vi "Write Current.vi"(8 "error in":errorcluster, 10 "Current":dbl, 11 "69X_79X in":refnum<class "7976A.lvclass">) -> (0 "error out":errorcluster, 3 "69X_79X out":refnum<class "7976A.lvclass">)   [LabVIEW 2019, in "7976A.lvlib" / "7976A.lvclass"]
uses:
  Library/7976A.lvclass
  C:/Users/Public/Documents/Development/builds/Instruments/PowerSupply.lvlibp/Library/PowerSupply.lvclass
  Library/7976A.lvclass/7976A.ctl
  Read Local Resource.vi
  builds/Instruments/PowerSupply.lvlibp/Library/PowerSupply.lvclass
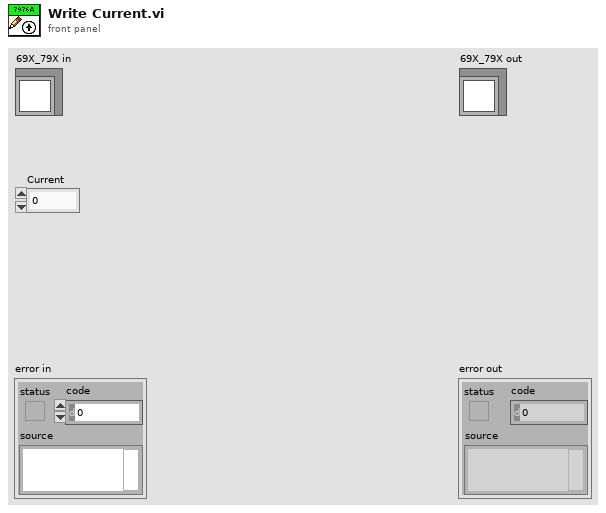
[diagram p1: front panel]
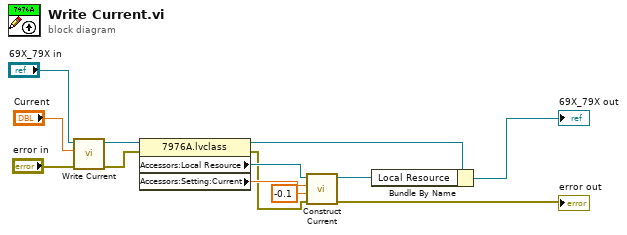
[diagram p0: block diagram]
diagram:
  n1 = call-parent "Write Current.vi"("error in"="error in", "Current"="Current", "PowerSupply in"="69X_79X in") -> ("error out"=w8:errorcluster, "PowerSupply out"=w10:refnum<class "7976A.lvclass">)  [unwired: 7 in]
  n2 = property class="7976A.lvclass"(reference=w10, error in=w8) -> (reference out=w9:refnum<class "7976A.lvclass">, error out=w3:errorcluster, "Accessors:Local Resource"=w6:refnum<visa-resource-name>, "Accessors:Setting:Current"=w5:dbl)
  n3 = call "Construct Current.vi"("error in (no error)"=w3, "Negative Current Limit"=-0.1, "Positive Current Limit"=w5, "VISA resource name"=w6) -> ("error out"=→"error out":errorcluster, "VISA resource name out"=w2:refnum<visa-resource-name>)  [unwired: 6 in]
  n4 = Bundle By Name(cluster=w9, "Local Resource"=w2) -> (→"69X_79X out":refnum<class "7976A.lvclass">)
